vi "Auto Json to cluster for step result.vi"(8 "error in (no error)":errorcluster, 11 "Message":string) -> (0 "error out":errorcluster, 3 "SEQ Status":T1 {"CMD" items=["Display Message", "Step Result", "Aborted", "Log Report", "Traceability", "Vision", "Seq Completed", "Print"]})   [LabVIEW 2017]
uses:
  controls/Seq Status to publish.ctl
  controls/Server CMDs to Publish.ctl
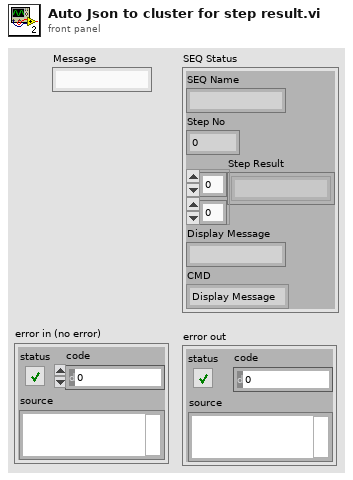
[diagram p1: front panel]
types:
  T1 = typedef "Seq Status to publish.ctl" = cluster{"SEQ Name":string, "Step No":i32, "Step Result":string[][], "Display Message":string, "CMD":T2}
  T2 = typedef "Server CMDs to Publish.ctl" = u16
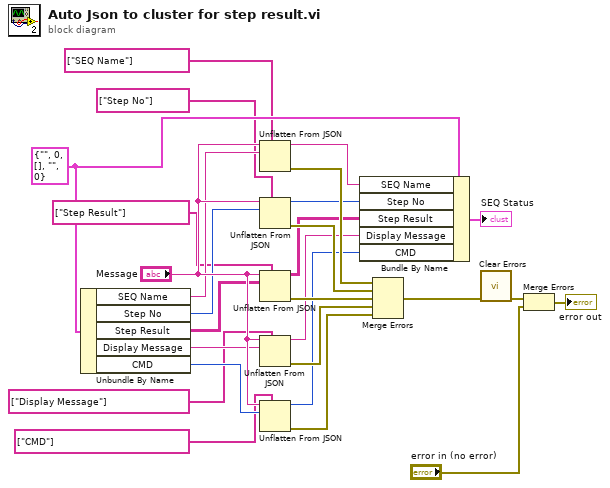
[diagram p0: block diagram]
diagram:
  w27 = T1 {"SEQ Name"="", "Step No"=0, "Step Result"=[], "Display Message"="", "CMD"=0} ("SEQ Status")
  n1 = Unbundle By Name(w27) -> ("SEQ Name"=w15:string, "Step No"=w16:i32, "Step Result"=w17:string[][], "Display Message"=w18:string, "CMD"=w20:T2)
  n2 = Unflatten From JSON(path=string[] ["SEQ Name"], JSON string="Message", type and defaults=w15) -> (value=w10:string, error out=w21:errorcluster)  [unwired: 4 in]
  n3 = Unflatten From JSON(path=string[] ["Step No"], JSON string="Message", type and defaults=w16) -> (value=w9:i32, error out=w22:errorcluster)  [unwired: 4 in]
  n4 = Unflatten From JSON(path=string[] ["Step Result"], JSON string="Message", type and defaults=w17) -> (value=w8:string[][], error out=w23:errorcluster)  [unwired: 4 in]
  n5 = Unflatten From JSON(path=string[] ["Display Message"], JSON string="Message", type and defaults=w18) -> (value=w7:string, error out=w24:errorcluster)  [unwired: 4 in]
  n6 = Unflatten From JSON(path=string[] ["CMD"], JSON string="Message", type and defaults=w20) -> (value=w6:T2, error out=w25:errorcluster)  [unwired: 4 in]
  n7 = Bundle By Name(cluster=w27, "SEQ Name"=w10, "Step No"=w9, "Step Result"=w8, "Display Message"=w7, "CMD"=w6) -> (→"SEQ Status":T1)
  n8 = Merge Errors(w21, w22, w23, w24, w25) -> (w26:errorcluster)
  n9 = call <vilib>:"Clear Errors.vi"("error in (no error)"=w26) -> ("error out"=w14:errorcluster)  [unwired: 5 in, 1 out]
  n10 = Merge Errors(w14, "error in (no error)") -> (→"error out":errorcluster)
